vi "测量处理数组数据的 VI 的运行时间.vi"() -> ()   [LabVIEW 2022 SP3]
panel:
  out "1~100累加":i32=33
  out "用时":dbl caption="Time to Match" format="%.3f"
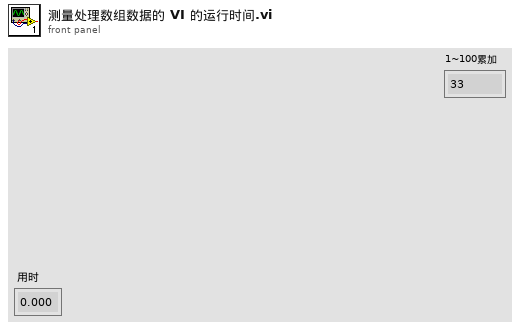
[diagram p1: front panel]
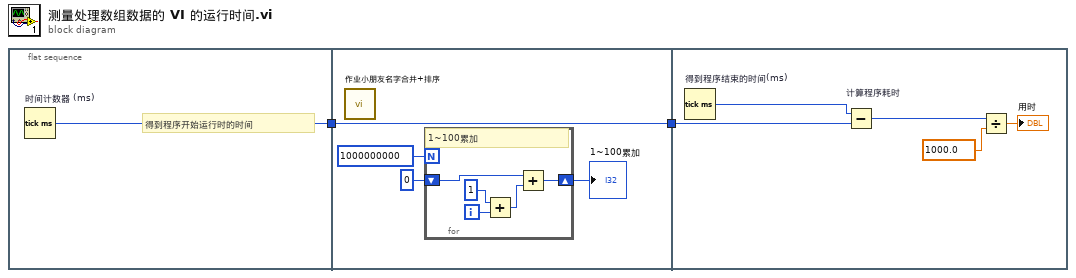
[diagram p0: block diagram]
diagram:
  n1 = flat-sequence {
    tunnel: [w3] -> w2
    tunnel: w2 -> [w7]
    tunnel: [w7] -> w1
    tunnel: w1 -> [w13]
    frame #0 {
      # "得到程序开始运行时的时间"
      n2 = Tick Count (ms) "时间计数器 (ms)"() -> (millisecond timer value=w3:u32)
    }
    frame #1 {
      n3 = call "作业小朋友名字合并+排序.vi"() -> ()  [unwired: 12 in]
      n4 = for {
        N: 1000000000 -> [_]
        shift-right: [w11] -> w6
        shift-left: 0 -> [w12]
        i -> [w9]
        # "1~100累加"
        n5 = Add(x=1, y=w9) -> (x+y=w8:i32)
        n6 = Add(x=w12, y=w8) -> (x+y=w11:i32)
      }
      "1~100累加" <- w6
    }
    frame #2 {
      n7 = Tick Count (ms) "得到程序结束的时间(ms)"() -> (millisecond timer value=w17:u32)
      n8 = Subtract "计算程序耗时"(x=w17, y=w13) -> (x-y=w16:u32)
      n9 = Divide(x=w16, y=1000.0) -> (x/y=→"用时":dbl)
    }
  }
